vi "Decoration - Free Label.vi"() -> ()   [LabVIEW 2016]
doc: "Sample numeric display item."
uses:
  <vilib>/NI Veristand/Display Template Support/Display Template Support.llb/cluster_Screen Item Settings.ctl
  <vilib>/NI Veristand/Display Template Support/Display Template Support.llb/cluster_Graph Scale Settings.ctl
  <vilib>/NI Veristand/Display Template Support/Display Template Support.llb/cluster_Graph Plot Settings.ctl
  <vilib>/NI Veristand/Display Template Support/Display Template Support.llb/enum_Display Template Handler Minimal To Widget Msg.ctl
  <vilib>/NI Veristand/Display Template Support/Display Template Support.llb/enum_Display Template Handler Minimal To Workspace.ctl
  <vilib>/NI Veristand/Display Template Support/Display Template Support.llb/sub_Display Template Handler Custom.vi
panel:
  in  "FreeText":string
  in  "Item.Data":T1
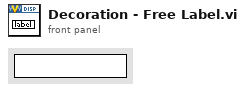
[diagram p1: front panel]
types:
  T1 = typedef "cluster_Screen Item Settings.ctl" = cluster{"Template VI":string, "Position X":i32, "Position Y":i32, "Custom":string, "Show Title Bar":bool, "ID":i32, "Always On Top":bool, "Allow Resize":bool, "Allow Minimize":bool, "Allow Close":bool, "Size to Screen":bool, "Screen.ID":i32, "State":enum16{"Normal", "New"}, "Title":string, "Window Bounds":cluster{"[0]":i16, "[1]":i16, "[2]":i16, "[3]":i16}, "Channel Ref":u64, "Unit":string, "Default Units?":bool, "Flash Limit?":bool, "Color 1":u32, "Color 2":u32, "Color 3":u32, "Color 4":u32, "Bck Color":u32, "Fore Color":u32, "Limit 1":dbl, "Limit 2":dbl, "Limit 3":dbl, "Limit 4":dbl, "Limit Mode 1":i32, "Limit Mode 2":i32, "Limit Mode 3":i32, "Limit Mode 4":i32, "Scale Precision":i32, "Scale Min":dbl, "Scale Max":dbl, "Format":i32, "Precision":i32, "Background Type":i32, "IDs":i32[], "Units":string[], "Labels":string[], "Scale Factor":dbl, "Scale Offset":dbl, "YScale Index":u32[], "XScale":T2, "YScales":T2[], "Plots":T3[], "Update Period":dbl, "History Length":dbl, "My.Ref":refnum<vi>, "Is Control?":bool, "Channel Paths":string[], "Custom Data":variant}
  T2 = typedef "cluster_Graph Scale Settings.ctl" = cluster{"Format":u8, "Precision":u8, "Fit":u8, "Label":string, "Use Default Label":bool, "Label Visible":bool, "Min":dbl, "Max":dbl}
  T3 = typedef "cluster_Graph Plot Settings.ctl" = cluster{"Bar Style":u8, "Fill To":i16, "Fill/PtColor":u32, "Line Style":u8, "Line Width":u8, "Color":u32, "Interp":u8, "Point Style":u8}
  T4 = typedef "enum_Display Template Handler Minimal To Workspace.ctl" = cluster{"Operation":enum16{"SetCustomData", "DeleteItem"}, "Data":variant}
  T5 = typedef "enum_Display Template Handler Minimal To Widget Msg.ctl" = enum16{"Stop", "LaunchConfigDialog"}
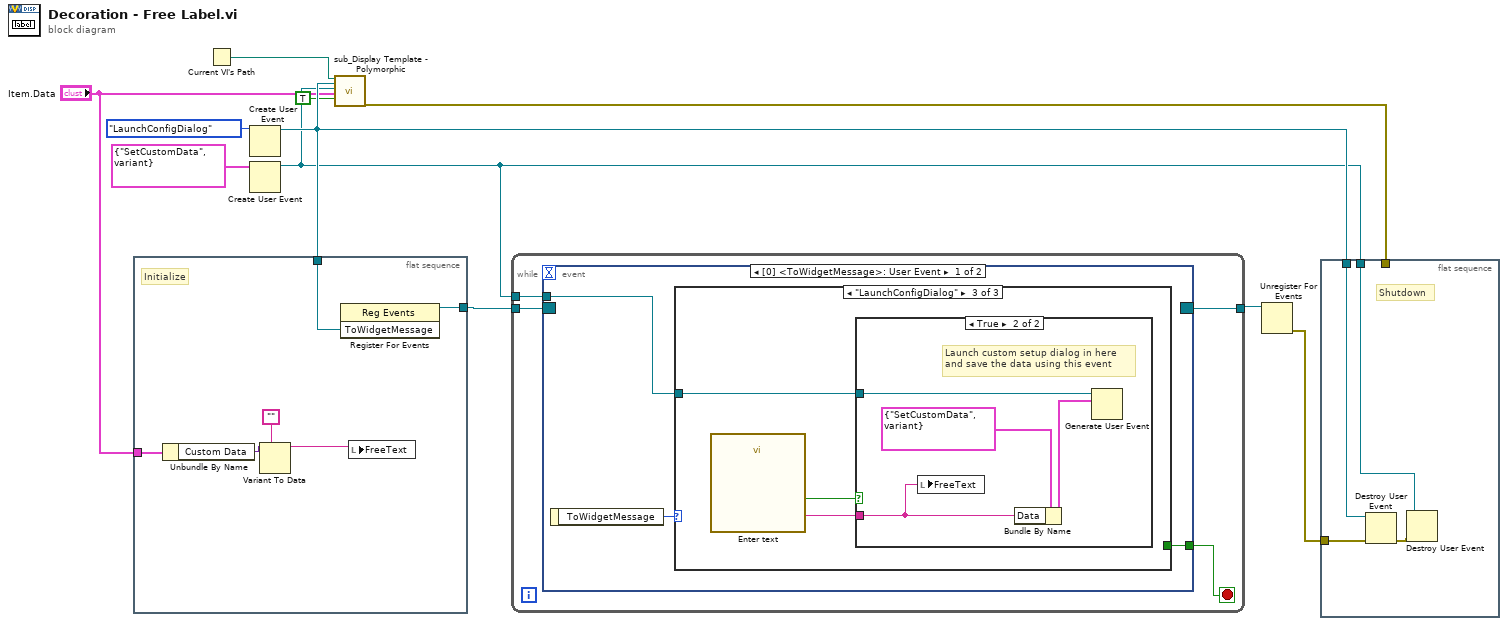
[diagram p0: block diagram]
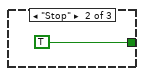
[diagram p3: hidden frame]
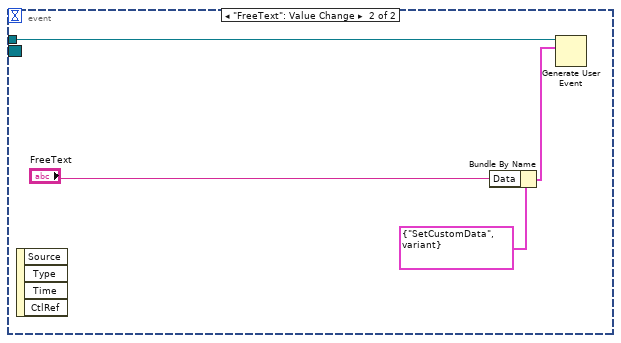
[diagram p5: hidden frame]
diagram:
  n1 = flat-sequence {
    tunnel: [w17] -> w9
    tunnel: w6 -> [w16]
    tunnel: "Item.Data" -> [w15]
    frame #0 {
      # "Initialize"
      n2 = Unbundle By Name(w15) -> ("Custom Data"=w14:variant)
      n3 = Variant To Data(type="", Variant=w14) -> (data=w12:string)  [unwired: 1 in, 1 out]
      n4 = register-events(w16) -> (reference out=w17:refnum<event-registration>)  [unwired: 2 in, 1 out]
      n5 = local write "FreeText"(w12) -> ()
    }
  }
  n6 = Current VI's Path() -> (path=w4:path)
  n7 = Create User Event(user event datatype=enum_Display_Template_Handler_Minimal_To_Widget_Msg."LaunchConfigDialog" ("ToWidgetMessage")) -> (user event=w6:refnum<user-event>)  [unwired: 1 in, 1 out]
  n8 = Create User Event(user event datatype=T4 {"Operation"=enum."SetCustomData", "Data"=variant} ("Data")) -> (user event=w2:refnum<user-event>)  [unwired: 1 in, 1 out]
  n9 = call-poly <vilib>:"sub_Display Template - Polymorphic.vi"("Parent.Path"=w4, "ToWidgetEvent"=w6, "ToWorkspace"=w2, "Item.Data"="Item.Data", "Resizable"=TRUE) -> ("error out"=w11:errorcluster)  [unwired: 1 in, 13 out]
  n10 = while {
    tunnel: w9 -> [w21]
    tunnel: [w19] -> w8
    tunnel: w2 -> [w18]
    stop <- w20 stop-if-true
    n11 = event shown="[0] <ToWidgetMessage>: User Event" {
      selector: w21 -> [_ _]
      dyn-events: [_ _] -> w19
      timeout: _ -> [_ _]
      tunnel: [w23 _] -> w20
      tunnel: w18 -> [w22 w36]
      event User Event {
        n12 = event-data() -> ("ToWidgetMessage"=w24:T5)  [unwired: 1 out]
        n13 = case shown="\"LaunchConfigDialog\"" w24 {
          tunnel: [_ TRUE _] -> w23
          tunnel: w22 -> [_ _ w28]
          frame Default {
          }
          frame "Stop" {
          }
          frame "LaunchConfigDialog" {
            n14 = call "Enter text"() -> ("Text"=w26:string, "OK"=w27:bool)  [unwired: 17 in, 1 out]
            n15 = case shown="True" w27 {
              tunnel: w28 -> [_ w32]
              tunnel: w26 -> [_ w29]
              frame False {
              }
              frame True {
                # "Launch custom setup dialog in here\nand save the data using this event"
                n16 = local write "FreeText"(w29) -> ()
                n17 = Bundle By Name(cluster=T4 {"Operation"=enum."SetCustomData", "Data"=variant} ("event data"), "Data"=w29) -> (w30:T4)
                n18 = Generate User Event(user event=w32, event data cluster=w30) -> ()  [unwired: 2 in, 2 out]
              }
            }
          }
        }
      }
      event "FreeText": Value Change {
        n19 = event-data() -> ()  [unwired: 5 out]
        n20 = Bundle By Name(cluster=T4 {"Operation"=enum."SetCustomData", "Data"=variant} ("event data"), "Data"="FreeText") -> (w33:T4)
        n21 = Generate User Event(user event=w36, event data cluster=w33) -> ()  [unwired: 2 in, 2 out]
      }
    }
  }
  n22 = Unregister For Events(event registration refnum=w8) -> (error out=w7:errorcluster)  [unwired: 1 in]
  n23 = flat-sequence {
    tunnel: w11 -> [_]
    tunnel: w7 -> [w39]
    tunnel: w6 -> [w40]
    tunnel: w2 -> [w37]
    frame #0 {
      # "Shutdown"
      n24 = Destroy User Event(user event=w40, error in=w39) -> (error out=w38:errorcluster)
      n25 = Destroy User Event(user event=w37, error in=w38) -> ()  [unwired: 1 out]
    }
  }
